vi "Start Command.vi"(8 "error in (no error)":errorcluster, 11 "Receiver Command in":refnum<class "Receiver Command.lvclass">) -> (0 "error out":errorcluster, 3 "Receiver Command out":refnum<class "Receiver Command.lvclass">)   [LabVIEW 2013, in "Receiver.lvlib" / "Receiver Commands Using Processor.lvlib" / "Receiver Command.lvclass"]
uses:
  Receiver Command.lvclass
  Command Processor/Command/Command.lvclass
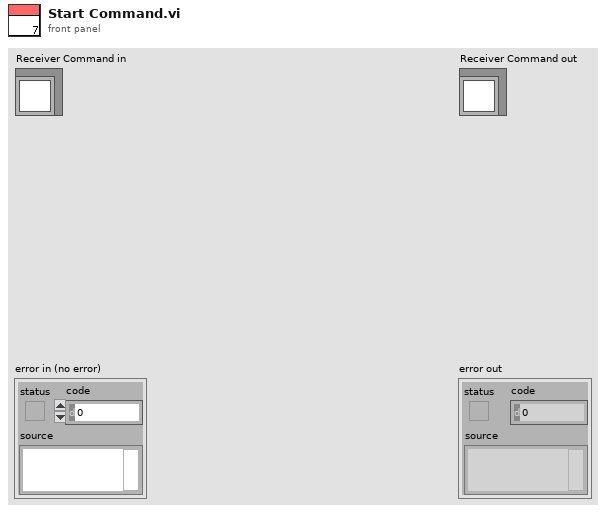
[diagram p1: front panel]
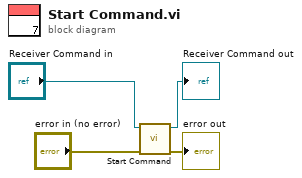
[diagram p0: block diagram]
diagram:
  n1 = call-parent "Start Command.vi"("error in (no error)"="error in (no error)", "Command in"="Receiver Command in") -> ("error out"=→"error out":errorcluster, "Command out"=→"Receiver Command out":refnum<class "Receiver Command.lvclass">)  [unwired: 8 in]
